vi "Close.vi"(8 "error in (no error)":errorcluster, 11 "uService Template in":refnum<class "Simple Device Manager.lvclass">) -> (0 "error out":errorcluster, 3 "uService Template out":refnum<class "Simple Device Manager.lvclass">)   [LabVIEW 2020, in "Simple Device Manager.lvlib" / "Simple Device Manager.lvclass"]
uses:
  Simple Device Manager.lvclass
  Simple Device Manager.lvclass/Simple Device Manager.ctl
  Hardware/Simple Device/Simple Device.lvclass
  TALOS/TALOS_PPL.lvlibp/Father of all uServices/Father of all uServices/Father of all uServices.lvclass
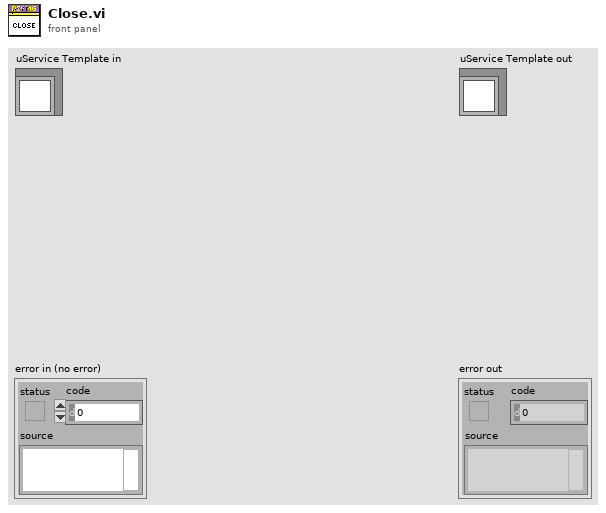
[diagram p1: front panel]
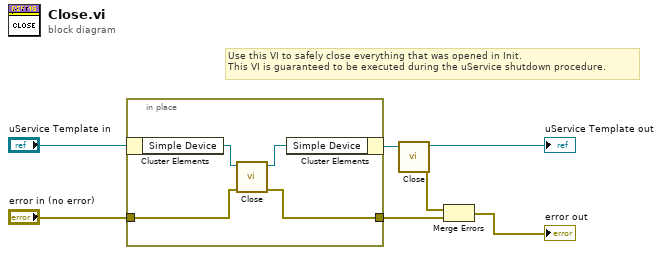
[diagram p0: block diagram]
diagram:
  # "Use this VI to safely close everything that was opened in Init.\nThis VI is guaranteed to be executed during the uService shutdown procedure."
  n1 = in-place {
    in-place-border: "error in (no error)" -> [w11]
    in-place-border: [w10] -> w3
    n2 = in-place-cluster #1("uService Template in") -> ("Simple Device"=w9:refnum<class "Simple Device.lvclass">)
    n3 = call-dynamic "Close.vi"("error in (no error)"=w11, "Simple Device in"=w9) -> ("error out"=w10:errorcluster, "Simple Device out"=w8:refnum<class "Simple Device.lvclass">)  [unwired: 8 in]
    n4 = in-place-cluster #1("Simple Device"=w8) -> (w1:refnum<class "Simple Device Manager.lvclass">)
  }
  n5 = call-parent "Close.vi"("uService Template in"=w1) -> ("error out"=w7:errorcluster, "uService Template out"=→"uService Template out":refnum<class "Simple Device Manager.lvclass">)  [unwired: 9 in]
  n6 = Merge Errors(w7, w3) -> (→"error out":errorcluster)
